vi "AI.Coupling.enum.convert.vi"(1 "AI.Coupling":T1=10050 items=["AC"=10045, "DC"=10050, "GND"=10066]) -> (0 "Numeric":i32)   [LabVIEW 2016, in "LockinDAQ.lvclass"]
uses:
  LockinDAQ.lvclass
  Typedefs/AI.coupling-enum.ctl
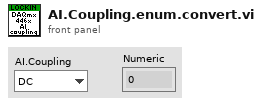
[diagram p1: front panel]
types:
  T1 = typedef "LockinDAQ.lvclass/AI.coupling-enum.ctl" = u16
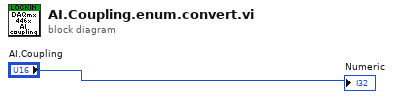
[diagram p0: block diagram]
diagram:
  "Numeric" <- "AI.Coupling"
